vi "Circle Coverage Score.vi"(10 "Rect Area":dbl, 11 "Radius":dbl) -> (3 "Score":dbl)   [LabVIEW 2015]
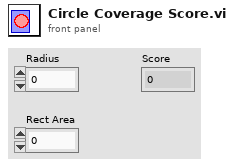
[diagram p1: front panel]
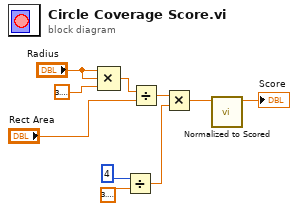
[diagram p0: block diagram]
diagram:
  n1 = Compound Arithmetic op=MULTIPLY("Radius", "Radius", 3.141592653589793) -> (w4:dbl)
  n2 = Divide(x=4 ("index (row)"), y=3.141592653589793) -> (x/y=w8:dbl)
  n3 = Divide(x=w4, y="Rect Area") -> (x/y=w7:dbl)
  n4 = Multiply(x=w7, y=w8) -> (x*y=w2:dbl)
  n5 = call "Normalized to Scored.vi"("Normalized in"=w2) -> ("Score out"=→"Score":dbl)  [unwired: 10 in]
